vi "DDS Com Check.vi"(4 "channel number (1)":u8=1 min=1 max=4 step=1, 6 "error in (no error)":errorcluster, 9 "DDS ref in":T1) -> (0 "error out":errorcluster, 2 "Passed?":bool, 3 "DDS ref out":T1)   [LabVIEW 2013]
doc: "Checks communication with the specified channel."
uses:
  DDS_box_device_reference.ctl
  <vilib>/ni845x/ni845x.llb/ni845xControl.ctl
  AD9910 registers.ctl
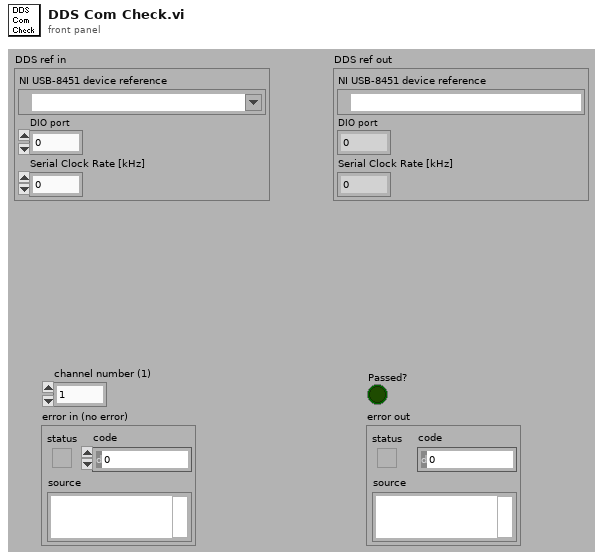
[diagram p1: front panel]
types:
  T1 = typedef "DDS_box_device_reference.ctl" = cluster{"NI USB-8451 device reference":T2, "DIO port":u8, "Serial Clock Rate [kHz]":u16}
  T2 = typedef "ni845xControl.ctl" = refnum<k21>
  T3 = typedef "AD9910 registers.ctl" = enum16{"CFR1", "CFR2", "CFR3", "Auxiliary DAC Control", "I/0 Update Rate", "Frequency Tuning Word", "Phase Offset Word", "Amplitude Scale Factor", "Multichip Sync", "Digital Ramp Limit", "Digital Ramp Step Size", "Digital Ramp Rate", "Single Tone Profile 0", "Single Tone Profile 1", "Single Tone Profile 2", "Single Tone Profile 3", "Single Tone Profile 4", "Single Tone Profile 5", "Single Tone Profile 6", "Single Tone Profile 7", "RAM Profile 0", "RAM Profile 1", "RAM Profile 2", "RAM Profile 3", "RAM Profile 4", "RAM Profile 5", "RAM Profile 6", "RAM Profile 7", "RAM"}
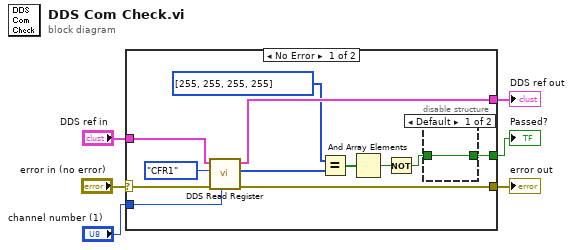
[diagram p0: block diagram]
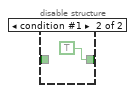
[diagram p2: hidden frame]
diagram:
  n1 = case shown="No Error" "error in (no error)" {
    selector: "error in (no error)" -> [w7 w21]
    tunnel: [w15 w22] -> w6
    tunnel: [w10 w21] -> w5
    tunnel: "DDS ref in" -> [w17 w22]
    tunnel: "channel number (1)" -> [w16 _]
    tunnel: [w9 _] -> w1
    frame No Error {
      n2 = call "DDS Read Register.vi"("channel number (1)"=w16, "error in (no error)"=w7, "Register"=AD9910_registers."CFR1", "DDS ref in"=w17) -> ("error out"=w10:errorcluster, "Read data"=w13:u8[], "DDS ref out"=w15:T1)  [unwired: 5 in]
      n3 = Equal?(x=u8[] [255, 255, 255, 255] ("Write Data"), y=w13) -> (x = y?=w12:bool[])
      n4 = And Array Elements(Boolean array=w12) -> (logical AND=w11:bool)
      n5 = Not(x=w11) -> (.not. x?=w8:bool)
      n6 = disable-structure shown="Default" {
        disable-tunnel: [w19 TRUE] -> w9
        disable-tunnel: w8 -> [w19 _]
        frame condition #0 (active) {
        }
        frame condition #1 {
        }
      }
    }
    frame Error {
    }
  }
  "DDS ref out" <- w6
  "error out" <- w5
  "Passed?" <- w1
